vi "Configure TX Bandwidth.vi"(8 "error in (no error)":errorcluster, 9 "Subcarrier Spacing (120 kHz)":T1=1 items=["60 kHz", "120 kHz"], 10 "Instance (1)":T2=1, 11 "VISA resource name":refnum<visa-resource-name>) -> (0 "error out":errorcluster, 3 "VISA resource name out":refnum<visa-resource-name>)   [LabVIEW 2015, in "Rohde&Schwarz CMXP NR FR2 Measurement.lvlib"]
doc: "Selects the subcarrier spacing for the measurement, for all carriers.\n\nAttribute:\nRSCMXPNRFR2M_ATTR_SUBCARRIER_SPACING\n\nRemote-control command:\nCONFigure:NRMMw:MEAS<i>:CCALl:TXBWidth:SCSPacing"
uses:
  <instrlib>/Rohde&Schwarz CMXP NR FR2 Measurement/Rohde&Schwarz CMXP NR FR2 Measurement.lvlib
  <instrlib>/Rohde&Schwarz CMXP NR FR2 Measurement/Private/_Instance.ctl
  <instrlib>/Rohde&Schwarz CMXP NR FR2 Measurement/Private/_Subcarrier Spacing.ctl
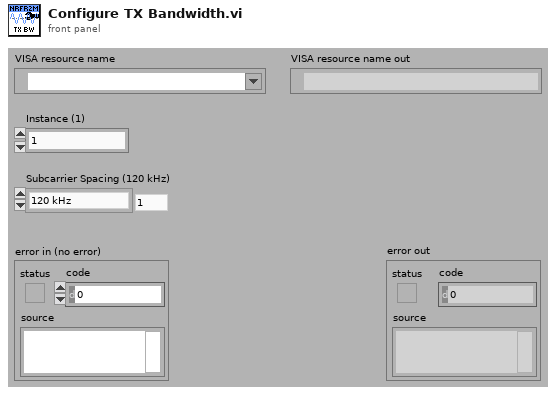
[diagram p1: front panel]
types:
  T1 = typedef "Rohde&Schwarz CMXP NR FR2 Measurement.lvlib/_Subcarrier Spacing.ctl" = i32
  T2 = typedef "Rohde&Schwarz CMXP NR FR2 Measurement.lvlib/_Instance.ctl" = i32
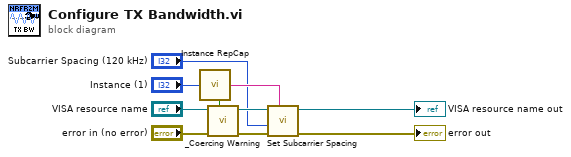
[diagram p0: block diagram]
diagram:
  n1 = call <instrlib>:"Instance RepCap.vi"("Instance In"="Instance (1)") -> ("In Range?"=w7:bool, "RepCap Identifier Out"=w3:string)  [unwired: 1 in]
  n2 = call <instrlib>:"_Coercing Warning.vi"("In Range?"=w7, "error in (no error)"="error in (no error)", "VISA resource name"="VISA resource name") -> ("error out"=w4:errorcluster, "VISA resource name out"=w5:refnum<visa-resource-name>)  [unwired: 7 in]
  n3 = call "Set Subcarrier Spacing"("Repeated Capabilities"=w3, "error in (no error)"=w4, "Subcarrier Spacing (0 - 60 kHz)"="Subcarrier Spacing (120 kHz)", "instrument handle"=w5) -> ("error out"=→"error out":errorcluster, "instrument handle out"=→"VISA resource name out":refnum<visa-resource-name>)  [unwired: 6 in]
